vi "Outputs.vi"(8 "error in (no error)":errorcluster, 11 "State in":T1={"State"=enum."Idle", "Start Time"=timestamp(0 s since 1904-01-01), "Configuration"={"DAQmx Task Name"="", "Output Channel"=0, "Time On (Sec)"=0.0, "Time Off (Sec)"=0.0, "Output Channel Names"=[], "Run?"=FALSE}, "Current Time"=timestamp(0 s since 1904-01-01), "First Iteration"=FALSE, "Data"={"D-O State"=0}, "Process Name"="", "Output Error"=FALSE, "Log Started"=FALSE} {"Data"."D-O State" items=["Default", "On", "Off", "Not Initialized"]}) -> (0 "error out":errorcluster, 3 "State out":T1={"State"=enum."Idle", "Start Time"=timestamp(0 s since 1904-01-01), "Configuration"={"DAQmx Task Name"="", "Output Channel"=0, "Time On (Sec)"=0.0, "Time Off (Sec)"=0.0, "Output Channel Names"=[], "Run?"=FALSE}, "Current Time"=timestamp(0 s since 1904-01-01), "First Iteration"=FALSE, "Data"={"D-O State"=0}, "Process Name"="", "Output Error"=FALSE, "Log Started"=FALSE} {"Data"."D-O State" items=["Default", "On", "Off", "Not Initialized"]})   [LabVIEW 2018, in "D-O Module.lvlib" / "D-O Module Engine.lvlib"]
uses:
  D-O Module Engine.lvlib
  Tag VIs/Tag FGV Operation Enum.ctl
  Shared Variables/Dynamic Shared Variables.lvlib
  <vilib>/DAQmx/write.llb/DAQmx Write (Digital Bool 1Line 1Point).vi
  DAQ/DAQ.lvlib
  Acquisition/Task Cluster.ctl
  Acquisition/Acquisition Settings Dialog.vi
  DAQ/DAQ Write Folder/DAQ/DAQ Write.lvlib
  support/Message Queue/Message Queue.lvlib
  support/Message Queue/Enqueue Message (Single).vi
  Acquisition/Acquisition State.ctl
  support/Message Queue/Message Cluster.ctl
  controls/Queue and Message Cluster.ctl
  <vilib>/Utility/error.llb/Error Cluster From Error Code.vi
  <vilib>/ErrorRing/Error Ring.xnode
  State Enum.ctl
  D-O Module Settings Cluster.ctl
  D-O Module.lvlib
  State Cluster.ctl
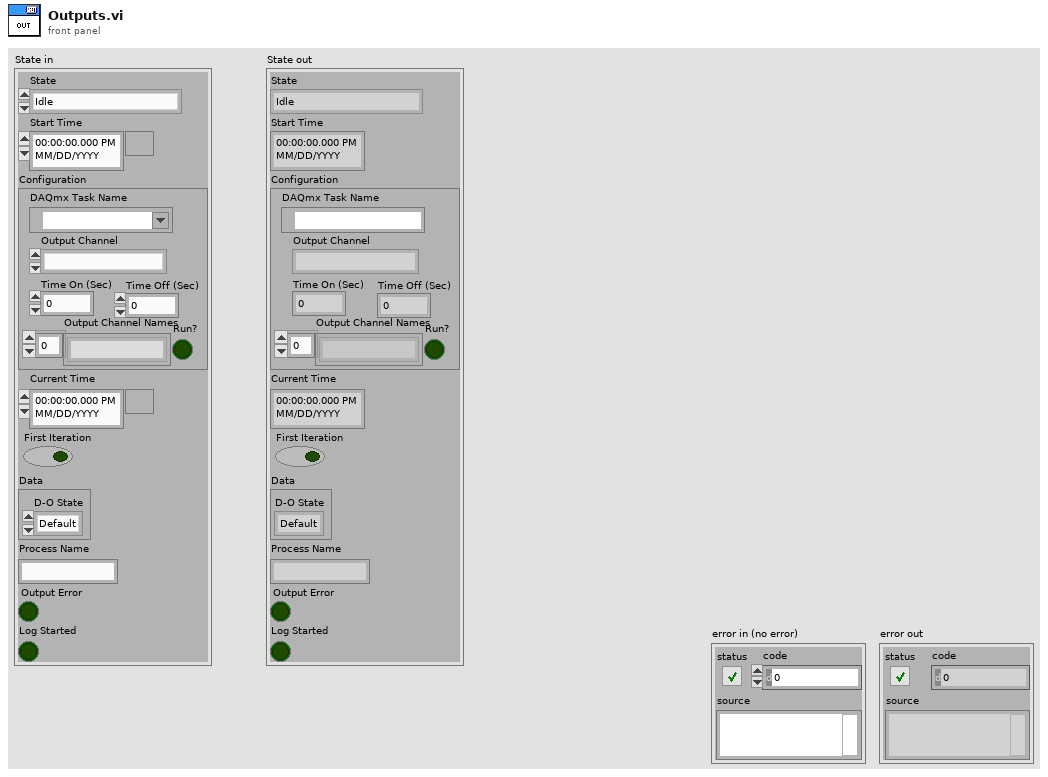
[diagram p1: front panel]
types:
  T1 = typedef "D-O Module.lvlib/D-O Module Engine.lvlib/State Cluster.ctl" = cluster{"State":T2, "Start Time":timestamp, "Configuration":T3, "Current Time":timestamp, "First Iteration":bool, "Data":cluster{"D-O State":u16}, "Process Name":string, "Output Error":bool, "Log Started":bool}
  T2 = typedef "D-O Module.lvlib/D-O Module Engine.lvlib/State Enum.ctl" = enum16{"Measuring", "Idle", "Paused"}
  T3 = typedef "D-O Module.lvlib/D-O Module Settings Cluster.ctl" = cluster{"DAQmx Task Name":refnum<k21>, "Output Channel":u16, "Time On (Sec)":dbl, "Time Off (Sec)":dbl, "Output Channel Names":string[], "Run?":bool}
  T4 = typedef "Tag FGV Operation Enum.ctl" = enum16{"Init", "Set Notification Queue", "Create Tag", "Commit", "Write Tag (Numeric)", "Write Tag (Boolean)", "Read All Tags", "Read One Tag", "Delete Tag Category", "Set Alarm Parameters (Numeric)", "Set Alarm Parameters (Boolean)", "Enable All Alarms", "Disable All Alarms", "Delete All Tags", "Read Alarms", "Ack Alarm"}
  T5 = typedef "D-O Module.lvlib/D-O Module Tag Names Cluster.ctl" = cluster{"D-O Status":string, "Output Device Tag":string}
  T6 = typedef "Task Cluster.ctl" = cluster{"DAQmx Task":refnum<k21>, "Read-Write Radio":enum32{"Read", "Write"}}
  T7 = typedef "DAQ Write.lvlib/Acquisition State.ctl" = enum16{"Idle", "Acquiring"}
  T8 = typedef "Queue and Message Cluster.ctl" = cluster{"return Message Queue":refnum<queue>, "Message":string, "Variant":variant}
  T9 = typedef "DAQ.lvlib/Hardware Configuration.ctl" = cluster{"Tasks":T6[]}
  T10 = typedef "Message Queue.lvlib/Message Cluster.ctl" = cluster{"Message":string, "Message Data":variant}
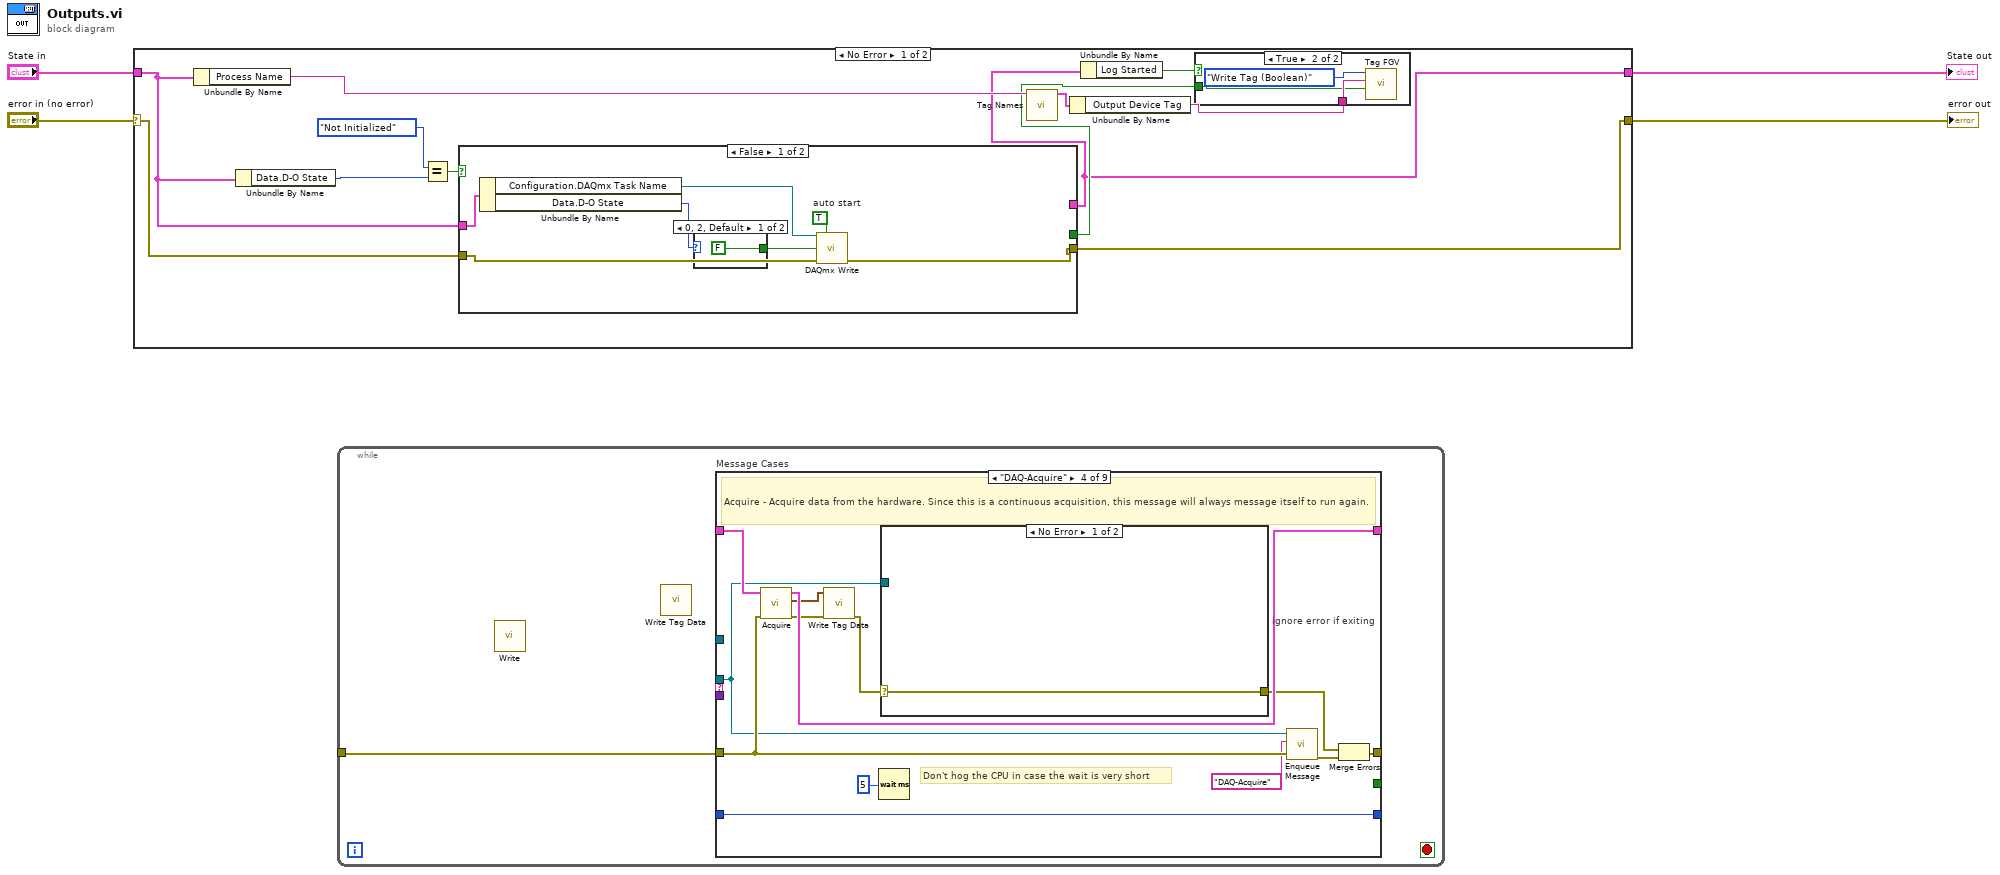
[diagram p0: block diagram]
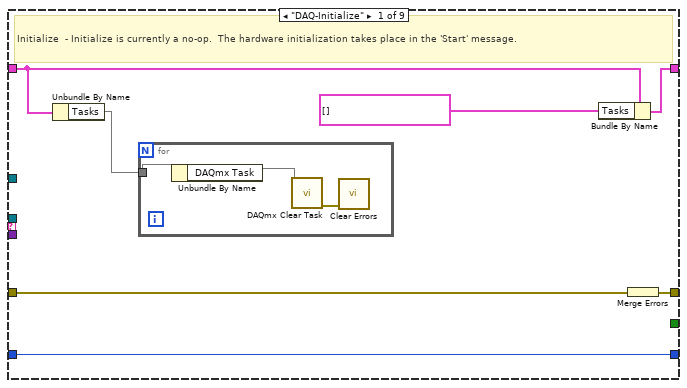
[diagram p2: hidden frame]
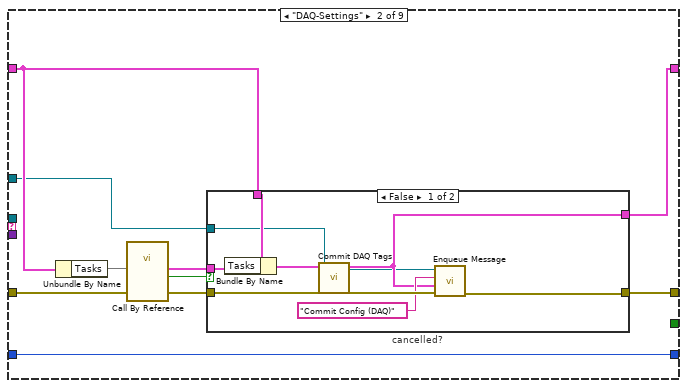
[diagram p3: hidden frame]
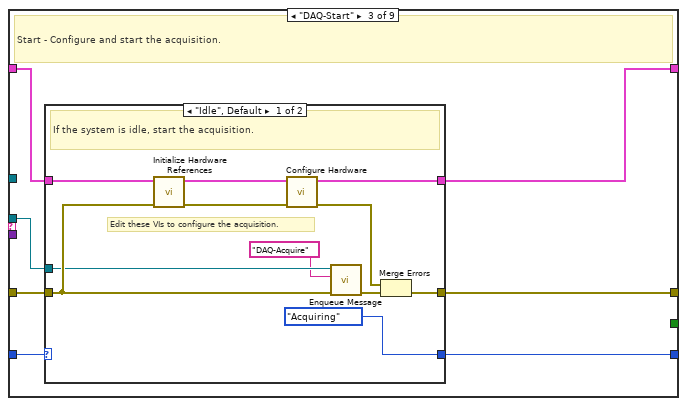
[diagram p5: hidden frame]
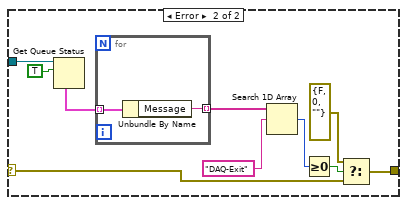
[diagram p7: hidden frame]
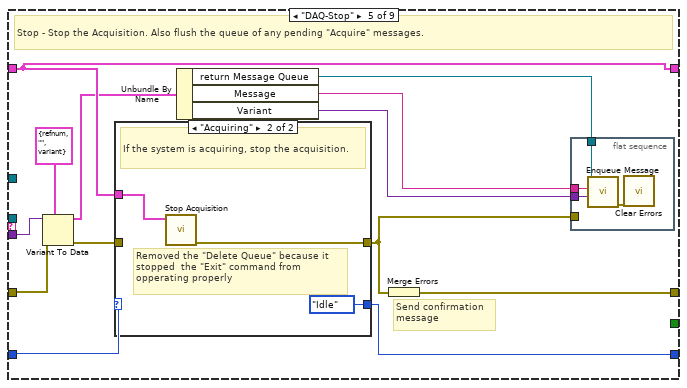
[diagram p8: hidden frame]
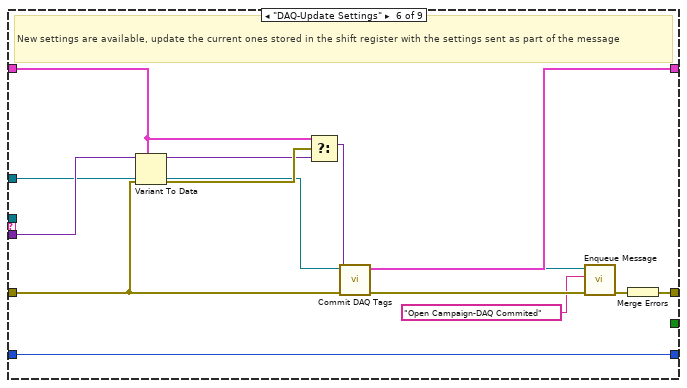
[diagram p10: hidden frame]
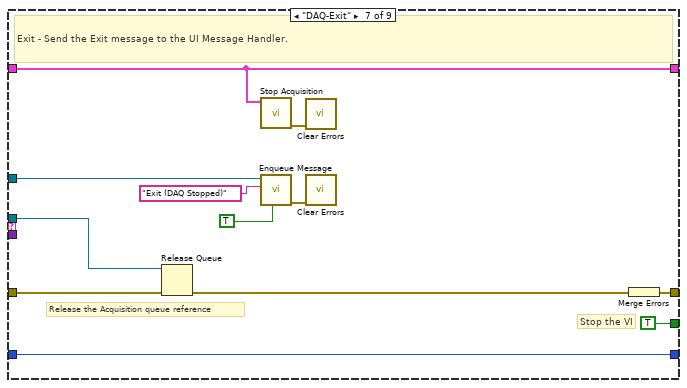
[diagram p11: hidden frame]
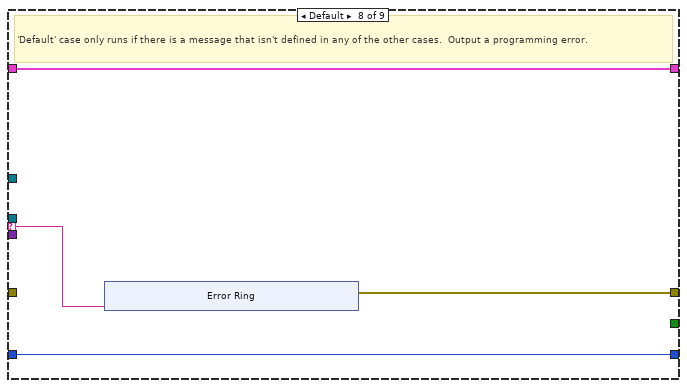
[diagram p12: hidden frame]
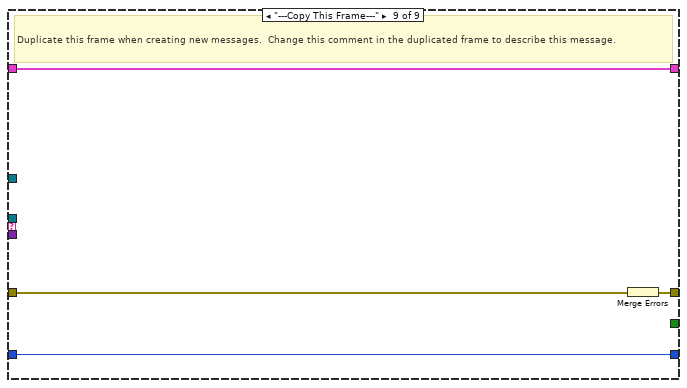
[diagram p13: hidden frame]
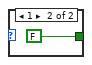
[diagram p15: hidden frame]
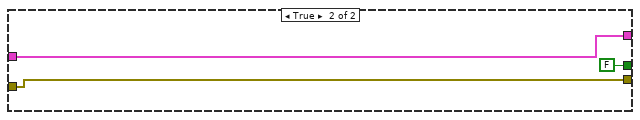
[diagram p16: hidden frame]
diagram:
  n1 = case shown="No Error" "error in (no error)" {
    selector: "error in (no error)" -> [w16 w33]
    tunnel: [w13 w33] -> w3
    tunnel: "State in" -> [w12 w32]
    tunnel: [w6 w32] -> w1
    frame No Error {
      n2 = Unbundle By Name(w12) -> ("Process Name"=w15:string)
      n3 = Unbundle By Name(w12) -> ("Data.D-O State"=w9:u16)
      n4 = Equal?(x=enum16{"Off", "On", "Not Initialized"}."Not Initialized", y=w9) -> (x = y?=w7:bool)
      n5 = case shown="False" w7 {
        tunnel: w16 -> [w21 w29]
        tunnel: [_ w30] -> w6
        tunnel: [w20 w29] -> w13
        tunnel: w12 -> [w26 w30]
        tunnel: [_ FALSE ("Connection Error")] -> w10
        frame False {
          w24 = TRUE  # auto start
          n6 = Unbundle By Name(w26) -> ("Configuration.DAQmx Task Name"=w23:refnum<k21>, "Data.D-O State"=w25:u16)
          n7 = case shown="0, 2, Default" w25 {
            tunnel: [FALSE ("D-O State") FALSE ("D-O State")] -> w22
            frame 0, 2, Default {
            }
            frame 1 {
            }
          }
          n8 = call-poly <vilib>:"DAQmx Write.vi"("task/channels in"=w23, "auto start"=w24, "data"=w22, "error in"=w21) -> ("error out"=w20:errorcluster)  [unwired: 9 in, 2 out]
        }
        frame True {
        }
      }
      n9 = call "Tag Names.vi"("Process Name"=w15) -> ("Pump Module Tag Names"=w14:T5)  [unwired: 8 in, 2 out]
      n10 = Unbundle By Name(w14) -> ("Output Device Tag"=w11:string)
      n11 = Unbundle By Name(w6) -> ("Log Started"=w5:bool)
      n12 = case shown="True" w5 {
        tunnel: w11 -> [_ w19]
        tunnel: w10 -> [_ w18]
        frame False {
        }
        frame True {
          n13 = call "Tag FGV.vi"("Data"=w18, "Tag Name"=w19, "Operation"=Tag_FGV_Operation_Enum."Write Tag (Boolean)") -> ()  [unwired: 3 in, 6 out]
        }
      }
    }
    frame Error {
    }
  }
  "error out" <- w3
  "State out" <- w1
  n14 = while {
    tunnel: _ -> [w34]
    stop <- _ stop-if-true
    n15 = call "Write.vi"() -> ()  [unwired: 10 in, 2 out]
    n16 = call "Write Tag Data.vi"() -> ()  [unwired: 9 in, 3 out]
    n17 = case "Message Cases" shown="\"DAQ-Acquire\"" {
      selector: _ -> [_ _ _ _ _ _ _ w162 _]
      tunnel: _ -> [_ _ w69 w89 _ _ w152 _ _]
      tunnel: w34 -> [w40 w52 w70 w97 w118 w139 w156 _ w174]
      tunnel: [w41 w46 w72 w99 w125 w147 w158 w161 w172] -> _
      tunnel: _ -> [w37 w50 w71 w95 w124 w143 w151 w163 w173]
      tunnel: [w38 w49 w68 w96 w124 w140 w151 w163 w173] -> _
      tunnel: [_ _ _ _ _ _ TRUE _ _] -> _
      tunnel: _ -> [_ _ _ _ w120 w146 _ _ _]
      tunnel: _ -> [_ w45 _ _ _ w136 w157 _ _]
      tunnel: _ -> [w39 w54 w67 w93 w123 w142 w150 w160 w171]
      tunnel: [w39 w54 w66 w93 w122 w142 w150 w160 w171] -> _
      frame "DAQ-Initialize" {
        # "Initialize  - Initialize is currently a no-op.  The hardware initialization takes place in the 'Start' message."
        n18 = Unbundle By Name(w37) -> ("Tasks"=w36)
        n19 = for {
          tunnel: w36 -> [w44]
          n20 = Unbundle By Name(w44) -> ("DAQmx Task"=w43)
          n21 = call <vilib>:"DAQmx Clear Task.vi"("task in"=w43) -> ("error out"=w42:errorcluster)  [unwired: 14 in]
          n22 = call <vilib>:"Clear Errors.vi"("error in (no error)"=w42) -> ()  [unwired: 5 in, 2 out]
        }
        n23 = Bundle By Name(cluster=w37, "Tasks"=T6[] []) -> (w38:cluster{})
        n24 = Merge Errors(w40) -> (w41:errorcluster)
      }
      frame "DAQ-Settings" {
        n25 = Unbundle By Name(w50) -> ("Tasks"=w51)
        n26 = call-by-ref "?"("error in (no error)"=w52, "Tasks in"=w51) -> ("error out"=w47:errorcluster, "cancelled"=w48:bool, "Tasks out"=w53:T6[])  [unwired: 9 in, 2 out]
        n27 = case "cancelled?" shown="False" w48 {
          tunnel: w53 -> [w63 _]
          tunnel: w50 -> [w62 w65]
          tunnel: [w57 w65] -> w49
          tunnel: w47 -> [w60 w64]
          tunnel: [w56 w64] -> w46
          tunnel: w45 -> [w55 _]
          frame False {
            n28 = Bundle By Name(cluster=w62, "Tasks"=w63) -> (w61:cluster{})
            n29 = call "Commit DAQ Tags.vi"("error in (no error)"=w60, "DAQ State in"=w61) -> ("error out"=w59:errorcluster, "DAQ State out"=w57:T9)  [unwired: 8 in]
            n30 = call-poly "Enqueue Message.vi"("error in (no error)"=w59, "Message Data"=w57, "Message"="Commit Config (DAQ)", "Message Queue"=w55) -> ("error out"=w56:errorcluster)  [unwired: 6 in, 1 out]
          }
          frame True {
          }
        }
      }
      frame "DAQ-Start" {
        # "Start - Configure and start the acquisition."
        n31 = case shown="\"Idle\", Default" w67 {
          selector: w67 -> [_ w84]
          tunnel: [w83 w86] -> w72
          tunnel: w71 -> [w82 w85]
          tunnel: w70 -> [w81 w86]
          tunnel: w69 -> [w79 _]
          tunnel: [w75 w85] -> w68
          tunnel: [Acquisition_State."Acquiring" ("State") w84] -> w66
          frame "Idle", Default {
            # "Edit these VIs to configure the acquisition."
            # "If the system is idle, start the acquisition."
            n32 = call "Initialize Hardware References.vi"("error in (no error)"=w81, "Hardware Resources in"=w82) -> ("error out"=w78:errorcluster, "Hardware Resources out"=w76:T9)  [unwired: 8 in]
            n33 = call "Configure Hardware.vi"("error in (no error)"=w78, "Hardware Resources in"=w76) -> ("error out"=w77:errorcluster, "Hardware Resources out"=w75:T9)  [unwired: 8 in]
            n34 = call-poly "Enqueue Message.vi"("error in (no error)"=w81, "Message"="DAQ-Acquire", "Message Queue"=w79) -> ("error out"=w80:errorcluster)  [unwired: 7 in, 1 out]
            n35 = Merge Errors(w77, w80) -> (w83:errorcluster)
          }
          frame "Acquiring" {
            # "The system is already acquiring. Ignore the \"Start\" message."
          }
        }
      }
      frame "DAQ-Acquire" {
        # "Don't hog the CPU in case the wait is very short"
        # "Acquire - Acquire data from the hardware. Since this is a continuous acquisition, this message will always message itself to run again."
        n36 = call "Acquire.vi"("error in (no error)"=w97, "Hardware Resources in"=w95) -> ("error out"=w92:errorcluster, "data"=w91:waveform(dbl)[], "Hardware Resources out"=w96:T9)  [unwired: 7 in]
        n37 = call "Write Tag Data.vi"("error in (no error)"=w92, "data"=w91) -> ("error out"=w88:errorcluster)  [unwired: 7 in, 2 out]
        n38 = Wait (ms)(milliseconds to wait=u32 5) -> ()  [unwired: 1 out]
        n39 = case "ignore error if exiting" shown="No Error" w88 {
          selector: w88 -> [w100 w103]
          tunnel: w89 -> [_ w110]
          tunnel: [w100 w102] -> w87
          frame No Error {
          }
          frame Error {
            n40 = Get Queue Status(queue=w110, return elements? (F)=TRUE) -> (elements=w107:T10[])  [unwired: 1 in, 7 out]
            n41 = for {
              tunnel: w107 -> [w112] mode=indexing
              tunnel: [w111] -> w106 mode=indexing
              n42 = Unbundle By Name(w112) -> ("Message"=w111:string)
            }
            n43 = Search 1D Array(1D array=w106, element="DAQ-Exit") -> (index of element=w105:i32)  [unwired: 1 in]
            n44 = Greater Or Equal To 0?(x=w105) -> (x >= 0?=w104:bool)
            n45 = Select(t=errorcluster {"status"=FALSE, "code"=0, "source"=""}, s=w104, f=w103) -> (s? t:f=w102:errorcluster)
          }
        }
        n46 = call-poly "Enqueue Message.vi"("error in (no error)"=w97, "Message"="DAQ-Acquire", "Message Queue"=w89) -> ("error out"=w98:errorcluster)  [unwired: 7 in, 1 out]
        n47 = Merge Errors(w87, w98) -> (w99:errorcluster)
      }
      frame "DAQ-Stop" {
        # "Send confirmation\nmessage"
        # "Stop - Stop the Acquisition. Also flush the queue of any pending \"Acquire\" messages."
        n48 = Variant To Data(error in=w118, type=T8 {"return Message Queue"=refnum, "Message"="", "Variant"=variant} ("Queue and Message"), Variant=w120) -> (data=w117:T8, error out=w119:errorcluster)
        n49 = case shown="\"Acquiring\"" w123 {
          selector: w123 -> [w131 _]
          tunnel: w119 -> [w130 _]
          tunnel: w124 -> [_ w134]
          tunnel: [w131 Acquisition_State."Idle" ("State")] -> w122
          tunnel: [w130 w132] -> w113
          frame "Idle", Default {
            # "The system is already idle. Ignore the \"Stop\" message."
          }
          frame "Acquiring" {
            # "Removed the \"Delete Queue\" because it\nstopped  the \"Exit\" command from \nopperating properly"
            # "If the system is acquiring, stop the acquisition."
            n50 = call "Stop Acquisition.vi"("Hardware Resources in"=w134) -> ("error out"=w132:errorcluster)  [unwired: 10 in]
          }
        }
        n51 = Unbundle By Name(w117) -> ("return Message Queue"=w116:refnum<queue>, "Message"=w115:string, "Variant"=w114:variant)
        n52 = Merge Errors(w113) -> (w125:errorcluster)
        n53 = flat-sequence {
          tunnel: w116 -> [w129]
          tunnel: w115 -> [w128]
          tunnel: w114 -> [w127]
          tunnel: w113 -> [_]
          frame #0 {
            n54 = call-poly "Enqueue Message.vi"("Message Data"=w127, "Message"=w128, "Message Queue"=w129) -> ("error out"=w126:errorcluster)  [unwired: 7 in, 1 out]
            n55 = call <vilib>:"Clear Errors.vi"("error in (no error)"=w126) -> ()  [unwired: 5 in, 2 out]
          }
        }
      }
      frame "DAQ-Update Settings" {
        # "New settings are available, update the current ones stored in the shift register with the settings sent as part of the message"
        n56 = Variant To Data(error in=w139, type=w143, Variant=w146) -> (data=w144:variant, error out=w145:errorcluster)
        n57 = Select(t=w143, s=w145, f=w144) -> (s? t:f=w141:variant)
        n58 = call "Commit DAQ Tags.vi"("error in (no error)"=w139, "DAQ State in"=w141) -> ("error out"=w138:errorcluster, "DAQ State out"=w140:T9)  [unwired: 8 in]
        n59 = call-poly "Enqueue Message.vi"("error in (no error)"=w138, "Message"="Open Campaign-DAQ Commited", "Message Queue"=w136) -> ("error out"=w137:errorcluster)  [unwired: 7 in, 1 out]
        n60 = Merge Errors(w137) -> (w147:errorcluster)
      }
      frame "DAQ-Exit" {
        # "Release the Acquisition queue reference"
        # "Stop the VI"
        # "Exit - Send the Exit message to the UI Message Handler."
        n61 = Release Queue(queue=w152, error in (no error)=w156) -> (error out=w153:errorcluster)  [unwired: 1 in, 2 out]
        n62 = call "Stop Acquisition.vi"("Hardware Resources in"=w151) -> ("error out"=w149:errorcluster)  [unwired: 10 in]
        n63 = call-poly "Enqueue Message.vi"("Priority Message? (F)"=TRUE, "Message"="Exit (DAQ Stopped)", "Message Queue"=w157) -> ("error out"=w148:errorcluster)  [unwired: 7 in, 1 out]
        n64 = call <vilib>:"Clear Errors.vi"("error in (no error)"=w149) -> ()  [unwired: 5 in, 2 out]
        n65 = call <vilib>:"Clear Errors.vi"("error in (no error)"=w148) -> ()  [unwired: 5 in, 2 out]
        n66 = Merge Errors(w153) -> (w158:errorcluster)
      }
      frame Default {
        # "'Default' case only runs if there is a message that isn't defined in any of the other cases.  Output a programming error."
        n67 = xnode "Error Ring"("parameter 0"=w162) -> ("error out"=w161:errorcluster)
      }
      frame "---Copy This Frame---" {
        # "Duplicate this frame when creating new messages.  Change this comment in the duplicated frame to describe this message."
        n68 = Merge Errors(w174) -> (w172:errorcluster)
      }
    }
  }
